vi "Parallel SR read.vi"(5 "Port Base Address":u32) -> (0 "Busy":bool, 1 "-Acknowledge":bool, 2 "Paper Empty":bool, 3 "Select":bool, 4 "-Error":bool)   [LabVIEW 2014]
doc: "Read from Status Register of Parallel Port\nThis VI determines the control register configuration of a parallel port. The four named bits may be low(F) or high(T). The Port Base Address should be the _base_ address; from there the VI gets the address of the control register itself.\nNote that this gets the actual output at the connector. You need not worry about the fact that for some bits the register is actually inverted relative to the output. This is separate from the fact that they may be 'active low'.\nThis VI uses the National Instruments AccessHW package to access the registers under Windows XP."
uses:
  <vilib>/Platform/portaccess.llb/In Port8.vi
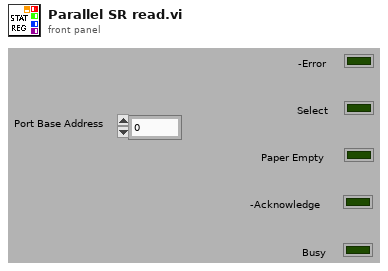
[diagram p1: front panel]
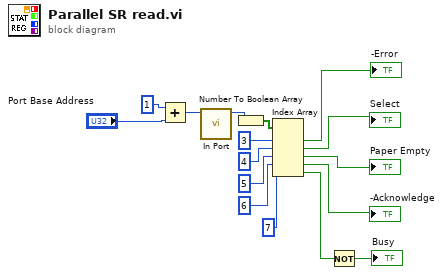
[diagram p0: block diagram]
diagram:
  n1 = Add(x=u32 1, y="Port Base Address") -> (x+y=w2:u32)
  n2 = call-poly <vilib>:"In Port.vi"("address"=w2) -> ("data read"=w1:i8)  [unwired: 7 in, 1 out]
  n3 = Number To Boolean Array(number=w1) -> (Boolean array=w14:bool[])
  n4 = Index Array(array=w14, index #1=3 ("index"), index #2=4 ("index"), index #3=5 ("index"), index #4=6 ("index"), index #5=7 ("index")) -> (element #1=→"-Error":bool, element #2=→"Select":bool, element #3=→"Paper Empty":bool, element #4=→"-Acknowledge":bool, element #5=w7:bool)
  n5 = Not(x=w7) -> (.not. x?=→"Busy":bool)
